vi "BLE_Module_EOL.vi"(0 "DUT":i32=1, 1 "DUTBLEName":string="MyESP32", 2 "DUTBLEMACAddress":string="d8:3b:da:49:e3:cd", 3 "Error In":errorcluster) -> (5 "Read Status":string, 7 "PASS":bool, 8 "FAIL":bool, 10 "Error Out":errorcluster)   [LabVIEW 2024]
doc: "Simple string based state machine with internal error handling.\n\n--------------------\n<Author>\n<Company>"
uses:
  controls/TypeDefReadBuffer.ctl
  controls/BLE_States.ctl
  <vilib>/Utility/error.llb/Trim Whitespace One-Sided.vi
  <vilib>/Instr/_visa.llb/VISA Configure Serial Port (Instr).vi
  Launcher/Launcher_DTU.lvlib
panel:
  out "read_buffer":T1
  in  "Stop":bool
  in  "VISA resource name":refnum<visa-resource-name>
  # "DTU1 macid:\nB4:77:45:4C:96:7C\n\nDTU2 macid:\nB4:77:45:4C:8E:A6"
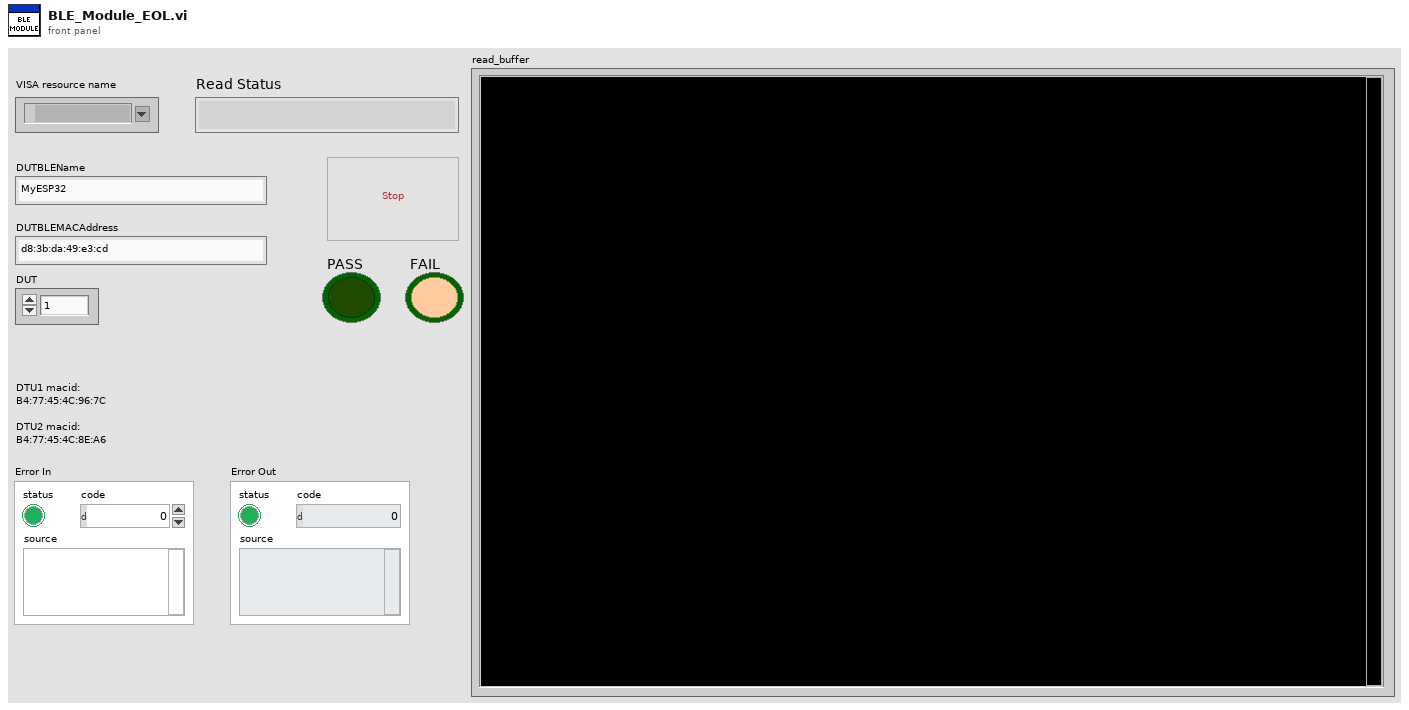
[diagram p1: front panel]
types:
  T1 = typedef "TypeDefReadBuffer.ctl" = string
  T2 = typedef "BLE_States.ctl" = enum16{"Init", "Init_BLE", "DUT_BLE_name", "DUT_BLE_macid", "scan", "ReadSerialContinously", "Disconnect_BLE", "Read_Disconnect_BLE", "Uninit_BLE", "Exit"}
  T3 = enum16{"Read", "Write", "All_sections", "All_values", "Remove key&section"}
  T4 = cluster{"Message":string, "VISA resource name":refnum<visa-resource-name>}
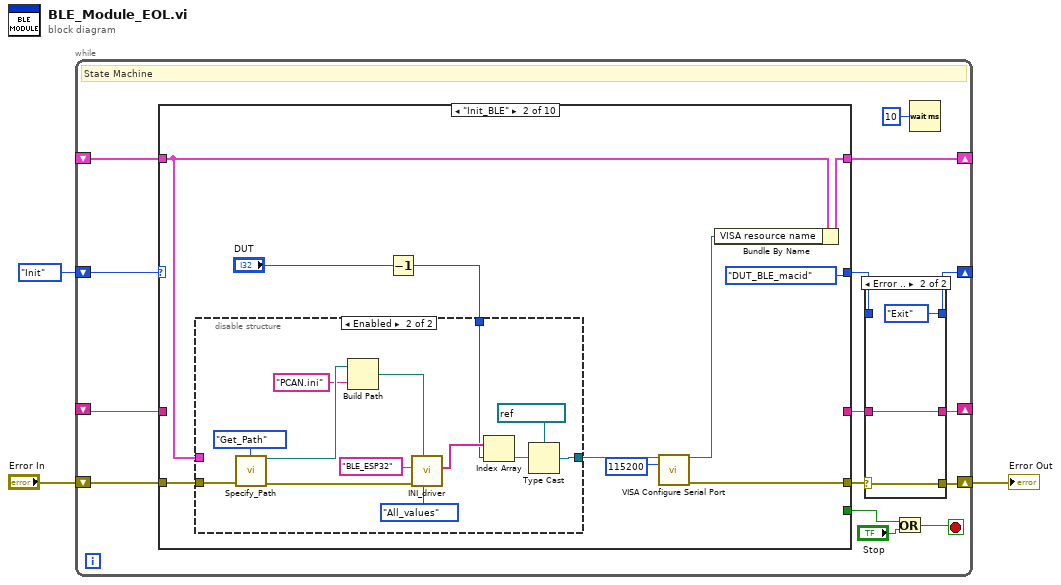
[diagram p0: block diagram]
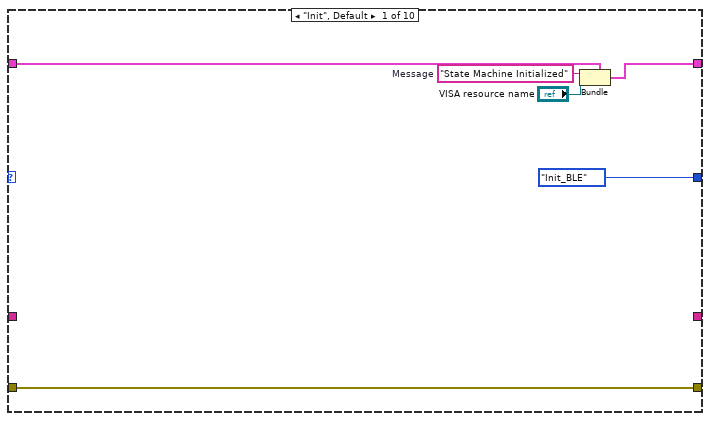
[diagram p2: hidden frame]
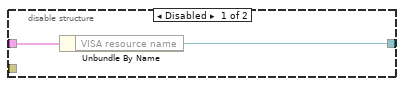
[diagram p3: hidden frame]
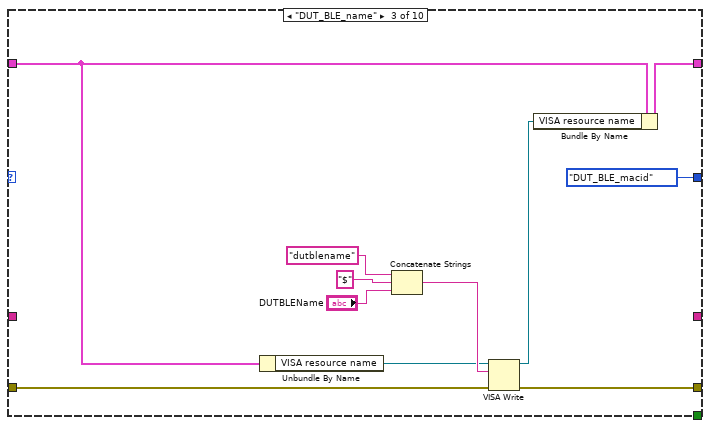
[diagram p4: hidden frame]
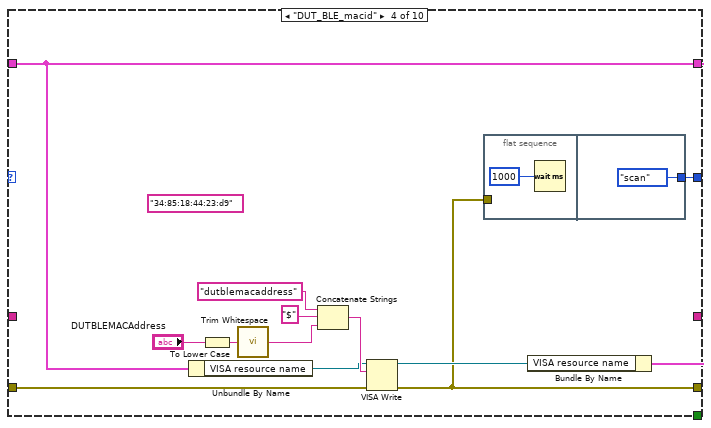
[diagram p5: hidden frame]
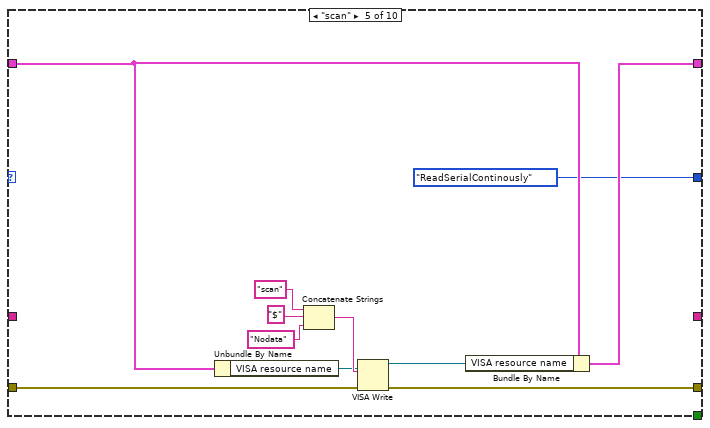
[diagram p6: hidden frame]
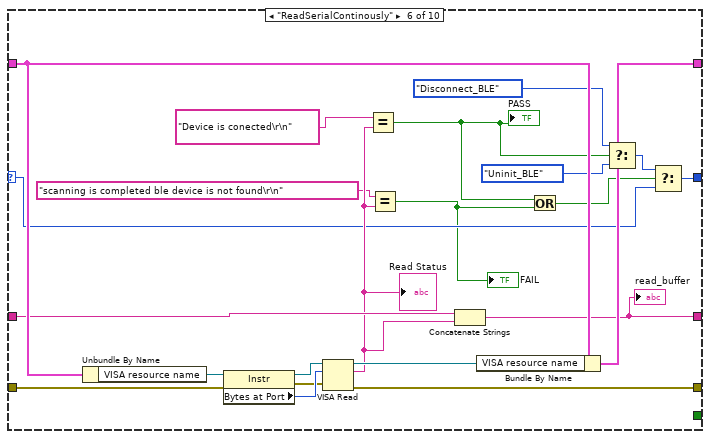
[diagram p7: hidden frame]
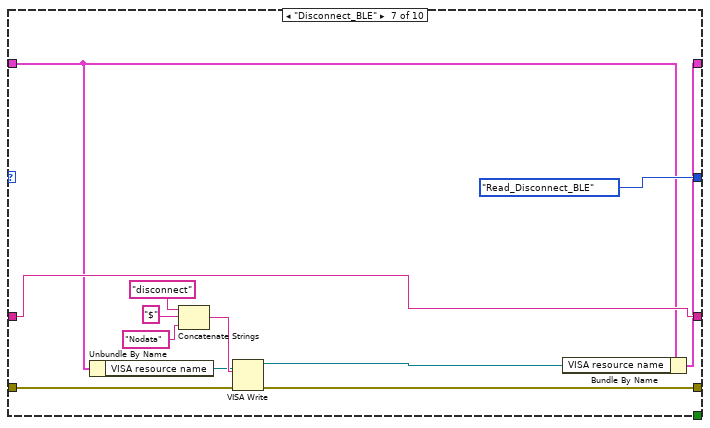
[diagram p8: hidden frame]
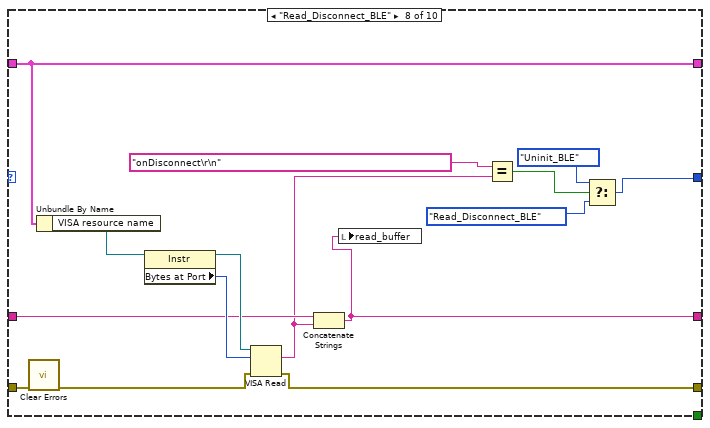
[diagram p9: hidden frame]
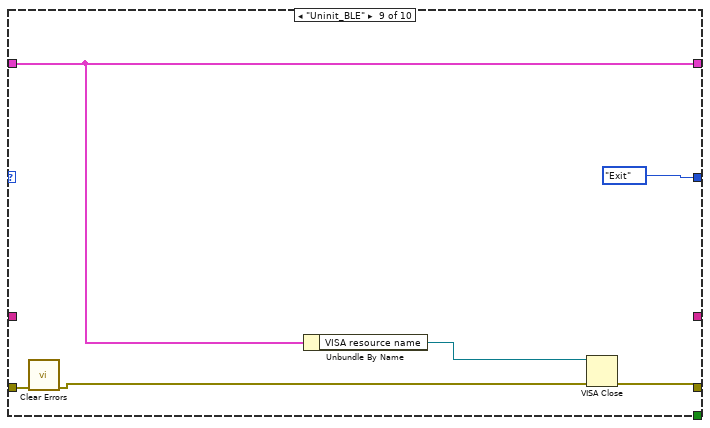
[diagram p10: hidden frame]
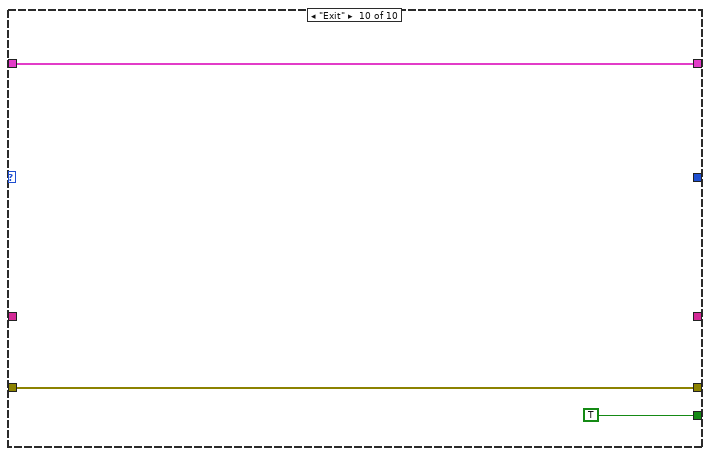
[diagram p11: hidden frame]
diagram:
  n1 = while {
    shift-right: [w11] -> _
    shift-left: BLE_States."Init" -> [w18]
    shift-right: [w16] -> _
    shift-left: _ -> [w17]
    shift-right: [w13] -> w3
    shift-left: "Error In" -> [w15]
    shift-right: [w5] -> _
    shift-left: _ -> [w6]
    stop <- w8 stop-if-true
    # "State Machine"
    n2 = case shown="\"Init_BLE\"" w18 {
      selector: w18 -> [_ _ _ _ _ w93 _ _ _ _]
      tunnel: w15 -> [w20 w27 w59 w71 w78 w104 w115 w134 w140 w142]
      tunnel: [w20 w33 w58 w64 w77 w108 w113 w127 w141 w142] -> w14
      tunnel: [_ _ _ _ _ _ _ _ _ TRUE] -> w9
      tunnel: [BLE_States."Init_BLE" BLE_States."DUT_BLE_macid" BLE_States."DUT_BLE_macid" w65 BLE_States."ReadSerialContinously" w98 BLE_States."Read_Disconnect_BLE" w124 BLE_States."Exit" _] -> w12
      tunnel: w17 -> [w21 w31 w53 w68 w80 w102 w111 w135 w137 w143]
      tunnel: [w23 w29 w51 w67 w79 w101 w109 w135 w137 w143] -> w16
      tunnel: w6 -> [_ _ _ _ _ w97 w112 w130 _ _]
      tunnel: [_ _ _ _ _ w96 w112 w129 _ _] -> w4
      frame "Init", Default {
        w24 = "State Machine Initialized"  # Message
        # "Initialize the state machine."
        n3 = Bundle(cluster=w21, "Message"=w24, "VISA resource name"="VISA resource name") -> (w23:T4)
      }
      frame "Init_BLE" {
        n4 = Decrement(x="DUT") -> (x-1=w25:i32)
        n5 = disable-structure shown="Enabled" {
          disable-tunnel: [w36 w37] -> w32
          disable-tunnel: w31 -> [w35 _]
          disable-tunnel: w27 -> [_ w46]
          disable-tunnel: w25 -> [_ w40]
          frame Disabled {
            n6 = Unbundle By Name(w35) -> ("VISA resource name"=w36:refnum<visa-resource-name>)
          }
          frame Enabled {
            n7 = call "Specify_Path.vi"("Path_Enum"=enum16{"Find_Path", "Get_Path"}."Get_Path", "error in (no error)"=w46) -> ("Configurations"=w44:path, "error out"=w48:errorcluster)  [unwired: 6 in, 6 out]
            n8 = Build Path(base path=w44, name or relative path="PCAN.ini") -> (appended path=w42:path)
            n9 = call "INI_driver.vi"("Enum"=T3."All_values", "instrument file path"=w42, "error in (no error)"=w48, "Section"="BLE_ESP32") -> ("Values out"=w41:string[])  [unwired: 4 in, 3 out]
            n10 = Index Array(array=w41, index=w40) -> (element=w39:string)
            n11 = Type Cast(type=refnum<visa-resource-name> "COM22" ("VISA resource name 2"), x=w39) -> (*(type *) &x=w37:refnum<visa-resource-name>)
          }
        }
        n12 = call-poly "VISA Configure Serial Port"("VISA resource name"=w32, "baud rate (9600)"=u32 115200) -> ("VISA resource name out"=w30:refnum<visa-resource-name>, "error out"=w33:errorcluster)  [unwired: 12 in]
        n13 = Bundle By Name(cluster=w31, "VISA resource name"=w30) -> (w29:T4)
      }
      frame "DUT_BLE_name" {
        n14 = Unbundle By Name(w53) -> ("VISA resource name"=w54:refnum<visa-resource-name>)
        n15 = Concatenate Strings("dutblename", "$" ("string"), "DUTBLEName") -> (w60:string)
        n16 = VISA Write(VISA resource name=w54, write buffer=w60, error in (no error)=w59) -> (VISA resource name out=w52:refnum<visa-resource-name>, error out=w58:errorcluster)  [unwired: 1 out]
        n17 = Bundle By Name(cluster=w53, "VISA resource name"=w52) -> (w51:T4)
      }
      frame "DUT_BLE_macid" {
        (unwired) "34:85:18:44:23:d9" ("DUTBLEMACAddress")
        n18 = Unbundle By Name(w68) -> ("VISA resource name"=w69:refnum<visa-resource-name>)
        n19 = To Lower Case(string="DUTBLEMACAddress") -> (all lower case string=w61:string)
        n20 = call <vilib>:"Trim Whitespace.vi"("string"=w61) -> ("trimmed string"=w62:string)  [unwired: 1 in]
        n21 = Concatenate Strings("dutblemacaddress", "$" ("string"), w62) -> (w70:string)
        n22 = VISA Write(VISA resource name=w69, write buffer=w70, error in (no error)=w71) -> (VISA resource name out=w66:refnum<visa-resource-name>, error out=w64:errorcluster)  [unwired: 1 out]
        n23 = flat-sequence {
          tunnel: w64 -> [_]
          tunnel: [BLE_States."scan"] -> w65
          frame #0 {
            n24 = Wait (ms)(milliseconds to wait=u32 1000) -> ()  [unwired: 1 out]
          }
          frame #1 {
          }
        }
        n25 = Bundle By Name(cluster=w68, "VISA resource name"=w66) -> (w67:T4)
      }
      frame "scan" {
        n26 = Unbundle By Name(w80) -> ("VISA resource name"=w82:refnum<visa-resource-name>)
        n27 = Concatenate Strings("scan", "$" ("string"), "Nodata" ("DUTBLEMACAddress 2")) -> (w83:string)
        n28 = VISA Write(VISA resource name=w82, write buffer=w83, error in (no error)=w78) -> (VISA resource name out=w81:refnum<visa-resource-name>, error out=w77:errorcluster)  [unwired: 1 out]
        n29 = Bundle By Name(cluster=w80, "VISA resource name"=w81) -> (w79:T4)
      }
      frame "ReadSerialContinously" {
        n30 = Unbundle By Name(w102) -> ("VISA resource name"=w107:refnum<visa-resource-name>)
        n31 = property class="Instr"(reference=w107, error in=w104) -> (reference out=w105:refnum<visa-resource-name>, error out=w103:errorcluster, "Bytes at Port"=w106:u32)
        n32 = VISA Read(VISA resource name=w105, byte count=w106, error in (no error)=w103) -> (VISA resource name out=w100:refnum<visa-resource-name>, read buffer=w95:string, error out=w108:errorcluster)  [unwired: 1 out]
        "Read Status" <- w95
        n33 = Equal?(x="Device is conected\r\n", y=w95) -> (x = y?=w88:bool)
        "PASS" <- w88
        n34 = Equal?(x="scanning is completed ble device is not found\r\n", y=w95) -> (x = y?=w87:bool)
        "FAIL" <- w87
        n35 = Concatenate Strings(w97, w95) -> (w96:string)
        "read_buffer" <- w96
        n36 = Bundle By Name(cluster=w102, "VISA resource name"=w100) -> (w101:T4)
        n37 = Or(x=w88, y=w87) -> (x .or. y?=w89:bool)
        n38 = Select(t=BLE_States."Disconnect_BLE", s=w88, f=BLE_States."Uninit_BLE" ("t")) -> (s? t:f=w90:T2)
        n39 = Select(t=w90, s=w89, f=w93) -> (s? t:f=w98:T2)
      }
      frame "Disconnect_BLE" {
        n40 = Unbundle By Name(w111) -> ("VISA resource name"=w116:refnum<visa-resource-name>)
        n41 = Concatenate Strings("disconnect", "$" ("string"), "Nodata" ("DUTBLEMACAddress 2")) -> (w117:string)
        n42 = VISA Write(VISA resource name=w116, write buffer=w117, error in (no error)=w115) -> (VISA resource name out=w110:refnum<visa-resource-name>, error out=w113:errorcluster)  [unwired: 1 out]
        n43 = Bundle By Name(cluster=w111, "VISA resource name"=w110) -> (w109:T4)
      }
      frame "Read_Disconnect_BLE" {
        # "Exit the State Machine"
        n44 = call <vilib>:"Clear Errors.vi"("error in (no error)"=w134) -> ("error out"=w128:errorcluster)  [unwired: 5 in, 1 out]
        n45 = Unbundle By Name(w135) -> ("VISA resource name"=w133:refnum<visa-resource-name>)
        n46 = property class="Instr"(reference=w133) -> (reference out=w132:refnum<visa-resource-name>, "Bytes at Port"=w131:u32)  [unwired: 1 in, 1 out]
        n47 = VISA Read(VISA resource name=w132, byte count=w131, error in (no error)=w128) -> (read buffer=w125:string, error out=w127:errorcluster)  [unwired: 2 out]
        n48 = Concatenate Strings(w130, w125) -> (w129:string)
        n49 = local write "read_buffer"(w129) -> ()
        n50 = Equal?(x="onDisconnect\r\n", y=w125) -> (x = y?=w123:bool)
        n51 = Select(t=BLE_States."Uninit_BLE", s=w123, f=BLE_States."Read_Disconnect_BLE") -> (s? t:f=w124:T2)
      }
      frame "Uninit_BLE" {
        # "Exit the State Machine"
        n52 = call <vilib>:"Clear Errors.vi"("error in (no error)"=w140) -> ("error out"=w139:errorcluster)  [unwired: 5 in, 1 out]
        n53 = Unbundle By Name(w137) -> ("VISA resource name"=w136:refnum<visa-resource-name>)
        n54 = VISA Close(VISA resource name=w136, error in (no error)=w139) -> (error out=w141:errorcluster)
      }
      frame "Exit" {
        # "Exit the State Machine"
      }
    }
    n55 = case shown="Error .." w14 {
      selector: w14 -> [w147 w150]
      tunnel: [w147 w150] -> w13
      tunnel: w12 -> [w146 _]
      tunnel: [w146 BLE_States."Exit"] -> w11
      tunnel: [w145 w148] -> w5
      tunnel: w4 -> [w145 w148]
      frame No Error {
      }
      frame Error {
      }
    }
    n56 = Or(x=w9, y="Stop") -> (x .or. y?=w8:bool)
    n57 = Wait (ms)(milliseconds to wait=u32 10) -> ()  [unwired: 1 out]
  }
  "Error Out" <- w3
